vi "Select Operation to Schedule Based on Rule.vi"(5 "EOJ":u16[](array[numeric]), 6 "Number of Machines":i32, 7 "Operation Selection Rule":T1=enum."SPT", 8 "Due Dates":u16[](array[numeric]), 9 "Processing Times":u16[][](array[numeric]), 10 "ES Subset":u16[](array[numeric]), 11 "Operation Subset":u16[](array[numeric])) -> (2 "Selected Operation's Start Time":u16, 3 "Selected Operation for Scheduling":u16)   [LabVIEW 2013, in "Scheduler.lvclass"]
uses:
  Scheduler.lvclass
  Operation Selection Rule from Subset to Schedule.ctl
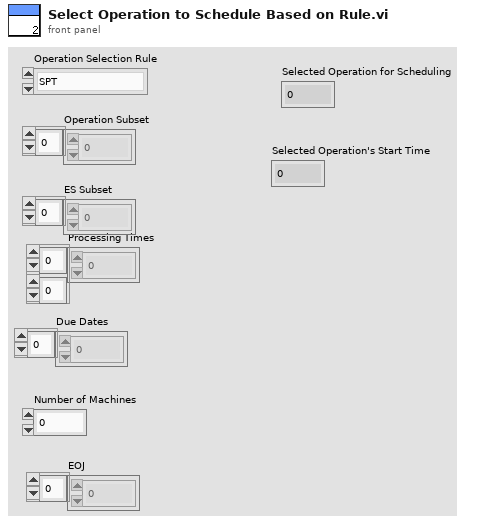
[diagram p1: front panel]
types:
  T1 = typedef "Scheduler.lvclass/Operation Selection Rule from Subset to Schedule.ctl" = enum16{"First Operation in Order", "SPT", "EDD", "MDD"}
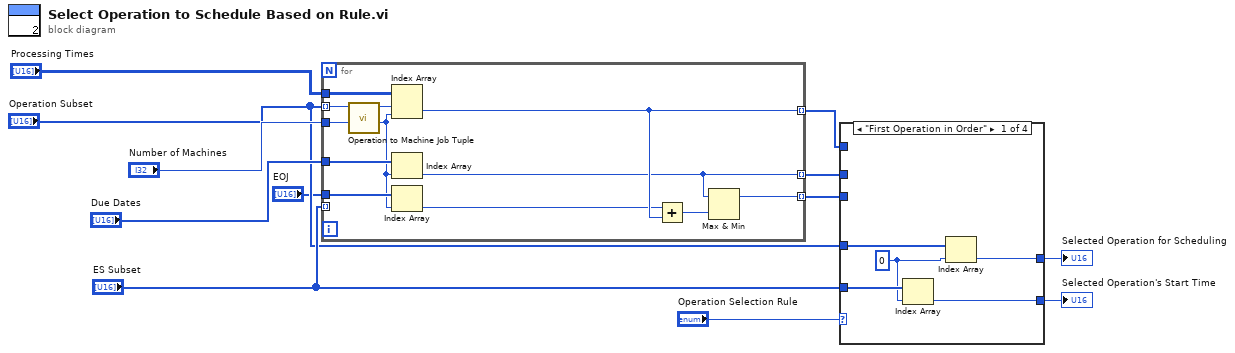
[diagram p0: block diagram]
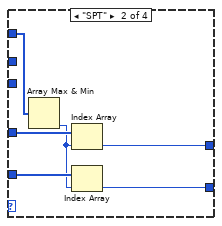
[diagram p2: hidden frame]
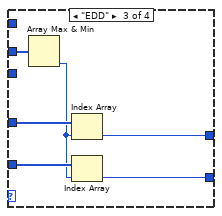
[diagram p3: hidden frame]
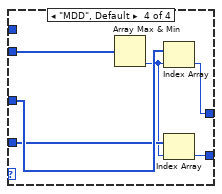
[diagram p4: hidden frame]
diagram:
  n1 = for {
    tunnel: "Operation Subset" -> [w24] mode=indexing
    tunnel: "Number of Machines" -> [w23]
    tunnel: "Processing Times" -> [w22]
    tunnel: [w19] -> w3 mode=indexing
    tunnel: "Due Dates" -> [w20]
    tunnel: [w17] -> w2 mode=indexing
    tunnel: [w16] -> w6 mode=indexing
    tunnel: "ES Subset" -> [_] mode=indexing
    tunnel: "EOJ" -> [w15]
    n2 = call "Operation to Machine Job Tuple.vi"("Number of Machines"=w23, "Operation Number"=w24) -> ("Job No"=w14:i32, "Machine No"=w21:i32)  [unwired: 8 in]
    n3 = Index Array(array=w22, index (row)=w21, index (col)=w14) -> (element=w19:u16)
    n4 = Index Array(array=w20, index=w14) -> (element=w17:u16)
    n5 = Index Array(array=w15, index=w14) -> (element=w13:u16)
    n6 = Add(x=w13, y=w19) -> (x+y=w18:u16)
    n7 = Max & Min(x=w17, y=w18) -> (max(x,y)=w16:u16)  [unwired: 1 out]
  }
  n8 = case shown="\"First Operation in Order\"" "Operation Selection Rule" {
    tunnel: w6 -> [_ _ _ w47]
    tunnel: "ES Subset" -> [w27 w32 w38 w45]
    tunnel: "Operation Subset" -> [w29 w34 w40 w46]
    tunnel: [w28 w33 w39 w43] -> w5
    tunnel: [w25 w30 w36 w42] -> w4
    tunnel: w3 -> [_ w35 _ _]
    tunnel: w2 -> [_ _ w41 _]
    frame "First Operation in Order" {
      w26 = 0 ("index")
      n9 = Index Array(array=w27, index=w26) -> (element=w25:u16)
      n10 = Index Array(array=w29, index=w26) -> (element=w28:u16)
    }
    frame "SPT" {
      n11 = Array Max & Min(array=w35) -> (min index (indices)=w31:i32)  [unwired: 3 out]
      n12 = Index Array(array=w34, index=w31) -> (element=w33:u16)
      n13 = Index Array(array=w32, index=w31) -> (element=w30:u16)
    }
    frame "EDD" {
      n14 = Array Max & Min(array=w41) -> (min index (indices)=w37:i32)  [unwired: 3 out]
      n15 = Index Array(array=w40, index=w37) -> (element=w39:u16)
      n16 = Index Array(array=w38, index=w37) -> (element=w36:u16)
    }
    frame "MDD", Default {
      n17 = Array Max & Min(array=w47) -> (min index (indices)=w44:i32)  [unwired: 3 out]
      n18 = Index Array(array=w46, index=w44) -> (element=w43:u16)
      n19 = Index Array(array=w45, index=w44) -> (element=w42:u16)
    }
  }
  "Selected Operation for Scheduling" <- w5
  "Selected Operation's Start Time" <- w4
